vi "Global variable.vi"() -> ()   [LabVIEW 2020]
panel:
  out "参数值记录":dbl[][](array[numeric])
  out "时间标识":timestamp
  out "数据":dbl[][](array[numeric])
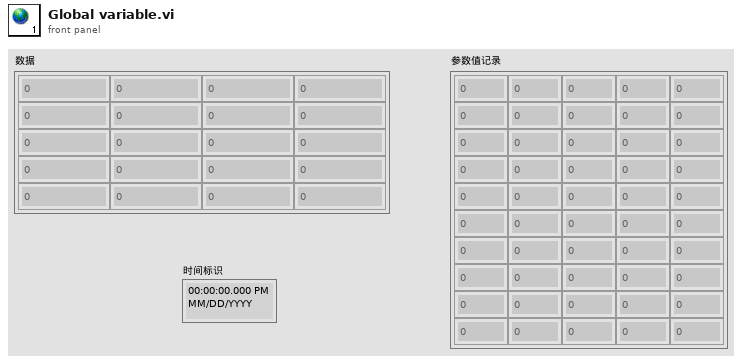
[diagram p1: front panel]
diagram:
